vi "SMGR_intercom_02.vi"(8 "error in (no error)":errorcluster, 10 "InputData":T1, 11 "URL:port":string="ssh.alwaysdata.com:12673") -> (0 "error out":errorcluster)   [LabVIEW 2010]
panel:
  out "FilePath":path
  out "FileType":string
  out "subarray 2":string[](array[string])
  out "subarray":string[](array[string])
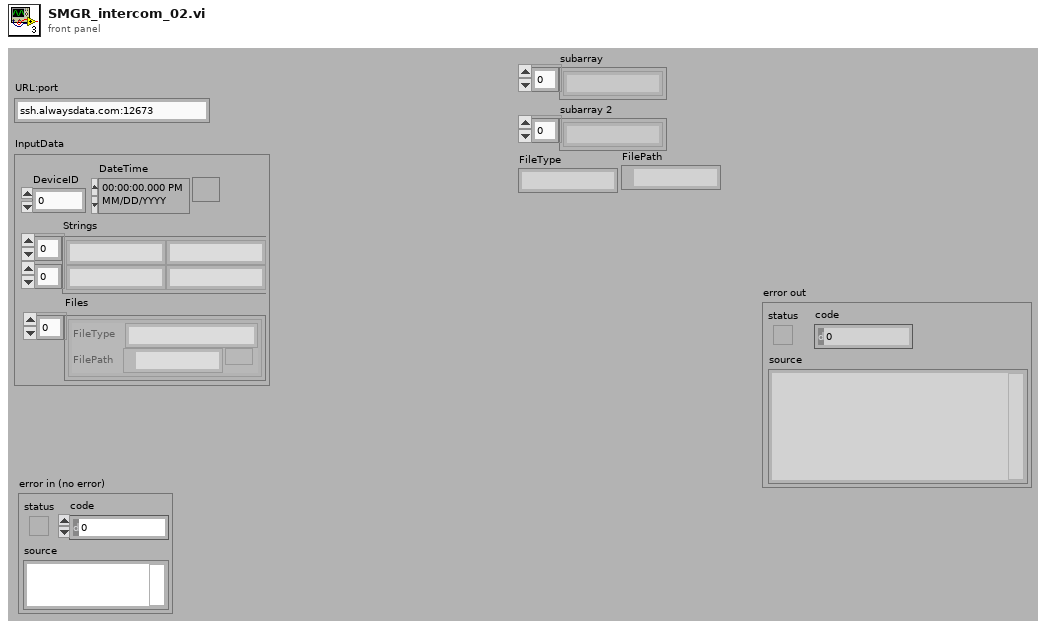
[diagram p1: front panel]
types:
  T1 = cluster{"DeviceID":i32, "DateTime":timestamp, "Files":cluster{"FileType":string, "FilePath":path}[], "Strings":string[][]}
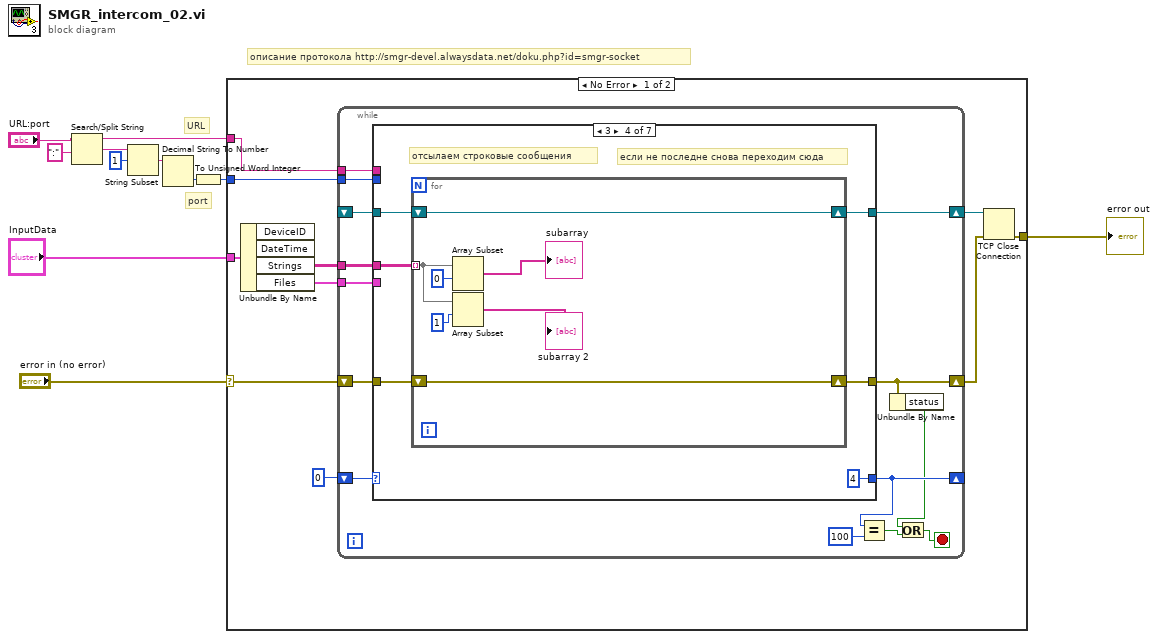
[diagram p0: block diagram]
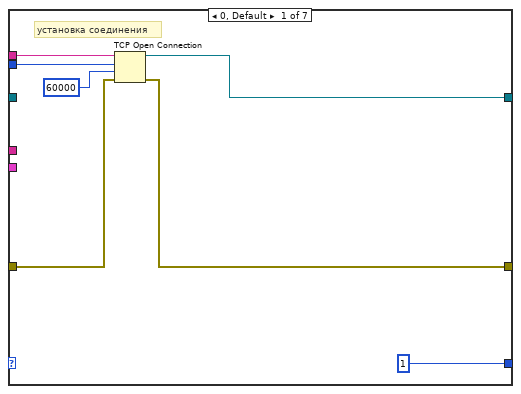
[diagram p2: hidden frame]
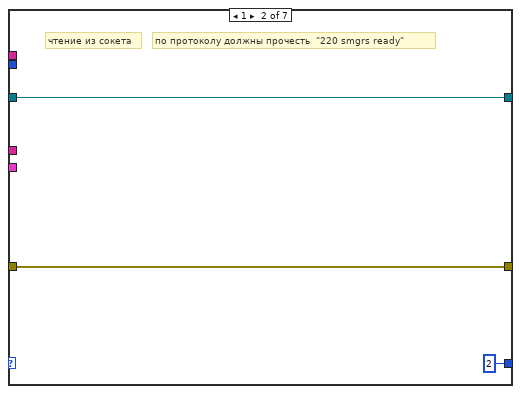
[diagram p3: hidden frame]
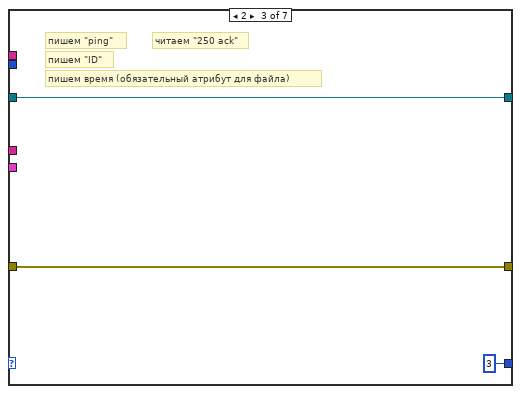
[diagram p4: hidden frame]
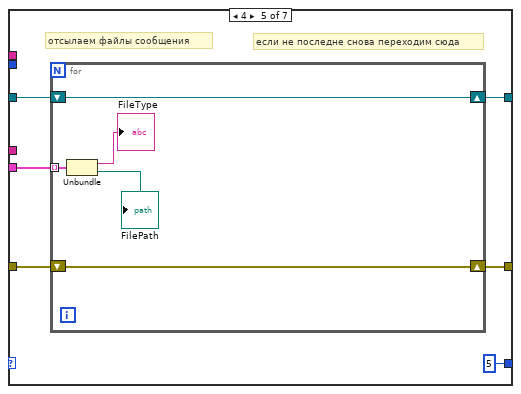
[diagram p5: hidden frame]
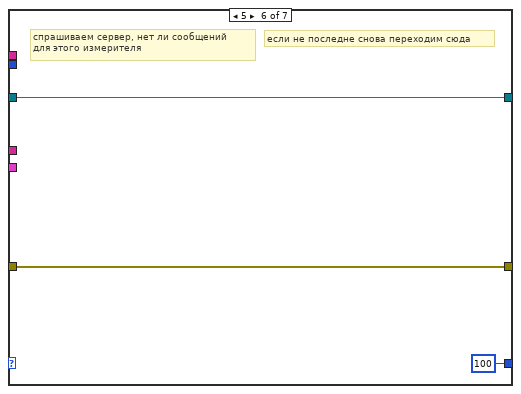
[diagram p6: hidden frame]
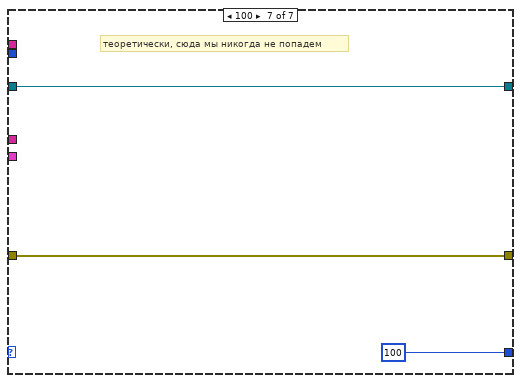
[diagram p7: hidden frame]
diagram:
  # "описание протокола http://smgr-devel.alwaysdata.net/doku.php?id=smgr-socket"
  # "port"
  # "URL"
  n1 = Search/Split String(string="URL:port", search string/char (-)=":") -> (substring before match=w5:string, match + rest of string=w8:string)  [unwired: 1 in, 1 out]
  n2 = String Subset(string=w8, offset (0)=1) -> (substring=w9:string)  [unwired: 1 in]
  n3 = Decimal String To Number(string=w9) -> (number=w4:i32)  [unwired: 2 in, 1 out]
  n4 = To Unsigned Word Integer(number=w4) -> (unsigned 16bit integer=w2:u16)
  n5 = case shown="No Error" "error in (no error)" {
    selector: "error in (no error)" -> [w20 w79]
    tunnel: w5 -> [w18 _]
    tunnel: w2 -> [w17 _]
    tunnel: "InputData" -> [w21 _]
    tunnel: [w14 w79] -> w1
    frame No Error {
      n6 = Unbundle By Name(w21) -> ("Strings"=w12:string[][], "Files"=w13:cluster{"FileType":string, "FilePath":path}[])  [unwired: 2 out]
      n7 = while {
        shift-right: [w28] -> _
        shift-left: 0 -> [w35]
        tunnel: w18 -> [w34]
        tunnel: w17 -> [w33]
        shift-right: [w25] -> w15
        shift-left: w20 -> [w32]
        shift-right: [w31] -> w16
        shift-left: _ -> [w30]
        tunnel: w12 -> [w23]
        tunnel: w13 -> [w22]
        stop <- w27 stop-if-true
        n8 = case shown="3" w35 {
          tunnel: [1 2 3 4 5 100 100] -> w28
          tunnel: w34 -> [w41 _ _ _ _ _ _]
          tunnel: w33 -> [w40 _ _ _ _ _ _]
          tunnel: w32 -> [w39 w45 w48 w52 w64 w75 w78]
          tunnel: [w38 w45 w48 w51 w63 w75 w78] -> w25
          tunnel: [w36 w43 w46 w49 w65 w73 w76] -> w31
          tunnel: w30 -> [_ w43 w46 w50 w66 w73 w76]
          tunnel: w23 -> [_ _ _ w53 _ _ _]
          tunnel: w22 -> [_ _ _ _ w62 _ _]
          frame 0, Default {
            # "установка соединения"
            n9 = TCP Open Connection(address=w41, remote port or service name=w40, timeout ms (60000)=60000, error in (no error)=w39) -> (connection ID=w36:refnum<k5>, error out=w38:errorcluster)  [unwired: 1 in]
          }
          frame 1 {
            # "по протоколу должны прочесть  \"220 smgrs ready\""
            # "чтение из сокета"
          }
          frame 2 {
            # "пишем время (обязательный атрибут для файла)"
            # "пишем \"ID\""
            # "читаем \"250 ack\""
            # "пишем \"ping\""
          }
          frame 3 {
            # "если не последне снова переходим сюда"
            # "отсылаем строковые сообщения"
            n10 = for {
              tunnel: w53 -> [w61] mode=indexing
              shift-right: [w59] -> w51
              shift-left: w52 -> [w59]
              shift-right: [w58] -> w49
              shift-left: w50 -> [w58]
              n11 = Array Subset(array=w61, index=0) -> (→"subarray":string[])  [unwired: 1 in]
              n12 = Array Subset(array=w61, index=1 ("length")) -> (→"subarray 2":string[])  [unwired: 1 in]
            }
          }
          frame 4 {
            # "если не последне снова переходим сюда"
            # "отсылаем файлы сообщения"
            n13 = for {
              tunnel: w62 -> [w70] mode=indexing
              shift-right: [w72] -> w63
              shift-left: w64 -> [w72]
              shift-right: [w71] -> w65
              shift-left: w66 -> [w71]
              n14 = Unbundle(w70) -> ("FileType"=→"FileType":string, "FilePath"=→"FilePath":path)
            }
          }
          frame 5 {
            # "если не последне снова переходим сюда"
            # "спрашиваем сервер, нет ли сообщений\nдля этого измерителя"
          }
          frame 100 {
            # "теоретически, сюда мы никогда не попадем"
          }
        }
        n15 = Equal?(x=w28, y=100) -> (x = y?=w26:bool)
        n16 = Unbundle By Name(w25) -> ("status"=w24:bool)
        n17 = Or(x=w24, y=w26) -> (x .or. y?=w27:bool)
      }
      n18 = TCP Close Connection(connection ID=w16, error in (no error)=w15) -> (error out=w14:errorcluster)  [unwired: 1 in, 1 out]
    }
    frame Error {
    }
  }
  "error out" <- w1
